vi "test_Double (Good).vi"(8 "error in (no error)":errorcluster, 11 "TestCase in":refnum<class "Test Read File.lvclass">) -> (0 "error out":errorcluster, 3 "TestCase out":refnum<class "Test Read File.lvclass">)   [LabVIEW 2019, in "Test Read File.lvclass"]
uses:
  Test Read File.lvclass
  C:/Program Files/National Instruments/LabVIEW 2024/vi.lib/Astemes/LUnit/Test Case.lvclass
  Test Read File.lvclass/Test Read File.ctl
  <vilib>/Astemes/LUnit/Test Case.lvclass/Test Case.ctl
  2e2e9b85-0683-485d-9539-f6f31d3c6460.vi
  <vilib>/Astemes/LUnit/Core/LUnit Test Case/Private/Append Pass Result.vi
  <vilib>/Astemes/LUnit/Core/LUnit Test Case/Private/Append Fail Result.vi
  2e2e9b85-0683-485d-9539-f6f31d3c6460.vi/9c5d11cd-9439-4240-a1ee-d9baace9c924.vi
  <vilib>/Astemes/LUnit/Core/LUnit Test Case/Private/Run In UI.vi
  <vilib>/Utility/error.llb/Clear Errors.vi
  Read/Read Section - Double.vi
  TSC File IO.lvlib
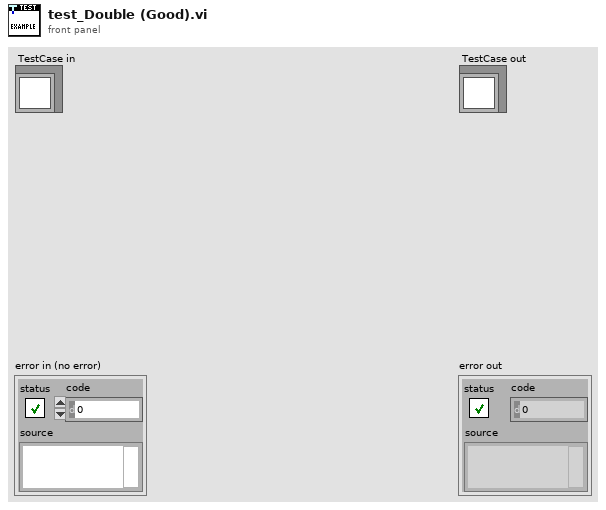
[diagram p1: front panel]
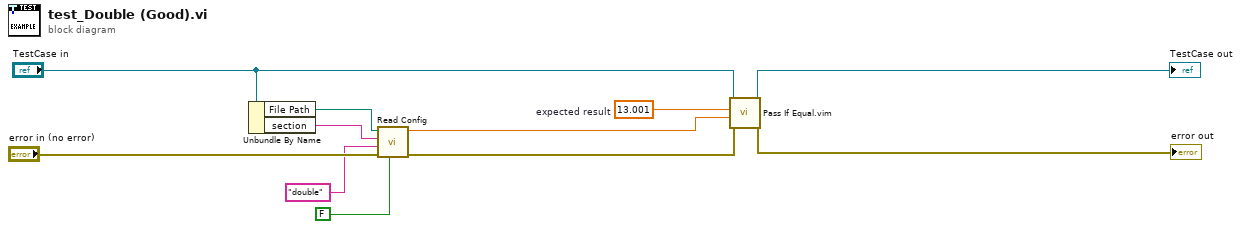
[diagram p0: block diagram]
diagram:
  w7 = 13.001  # expected result
  n1 = Unbundle By Name("TestCase in") -> ("File Path"=w5:path, "section"=w4:string)
  n2 = call-poly "Read Config.vi"("Create file if not found? (T)"=FALSE, "error in (no error)"="error in (no error)", "key"="double", "section"=w4, "Path"=w5) -> ("error out"=w6:errorcluster, "value"=w3:dbl)  [unwired: 5 in]
  n3 = call "Pass If Equal.vim"("error in (no error)"=w6, "Actual"=w3, "Expected"=w7, "LUnit Test Case In"="TestCase in") -> ("error out"=→"error out":errorcluster, "LUnit Test Case Out"=→"TestCase out":refnum<class "Test Read File.lvclass">)  [unwired: 6 in]
